vi "Set Torque Setpoint.vi"(8 "error in (no error)":errorcluster, 10 "current (A)":dbl, 11 "NI_Robotics_KUKA youBot Arm Motor_EtherCAT in":refnum<class "NI_Robotics_KUKA youBot Arm Motor_EtherCAT.lvclass">) -> (0 "error out":errorcluster, 3 "NI_Robotics_KUKA youBot Arm Motor_EtherCAT out":refnum<class "NI_Robotics_KUKA youBot Arm Motor_EtherCAT.lvclass">)   [LabVIEW 2017, in "NI_Robotics_KUKA youBot Host.lvlib" / "NI_Robotics_KUKA youBot Arm Motor_EtherCAT.lvclass"]
uses:
  <vilib>/robotics/KUKA youBot/Motor/Arm Motor EtherCAT/NI_Robotics_KUKA youBot Arm Motor_EtherCAT.lvclass
  <vilib>/robotics/KUKA youBot/Motor/Arm Motor EtherCAT/NI_Robotics_KUKA youBot Arm Motor_EtherCAT.lvclass/NI_Robotics_KUKA youBot Arm Motor_EtherCAT.ctl
  <vilib>/robotics/KUKA youBot/EtherCAT/Control Mode.ctl
  <vilib>/robotics/KUKA youBot/NI_Robotics_KUKA youBot Host.lvlib
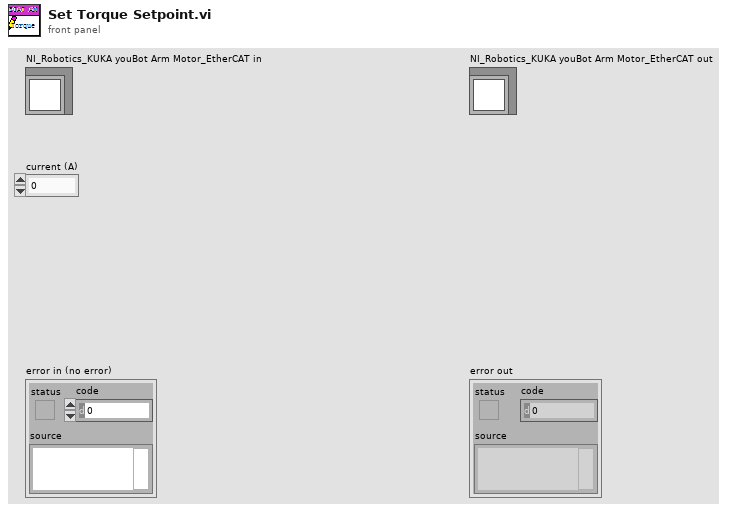
[diagram p1: front panel]
types:
  T1 = typedef "NI_Robotics_KUKA youBot Host.lvlib/Control Mode.ctl" = u8
  T2 = typedef "NI_Robotics_KUKA youBot Host.lvlib/Motor Slave Info.ctl" = cluster{"controller mode var":refnum<k21>, "reference var":refnum<k21>, "current var":refnum<k21>, "velocity var":refnum<k21>, "position var":refnum<k21>, "status var":refnum<k21>, "valid":bool, "status var type":enum16{"Int16", "Int32"}, "nodeAddr":u16, "masterHdl":T3}
  T3 = typedef "NI_Robotics_KUKA youBot Host.lvlib/Mater Handler.ctl" = i32
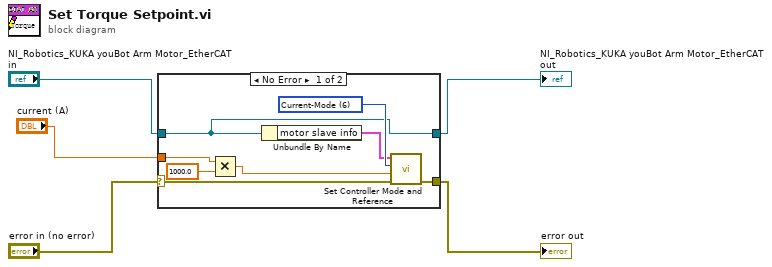
[diagram p0: block diagram]
diagram:
  n1 = case shown="No Error" "error in (no error)" {
    selector: "error in (no error)" -> [w9 w14]
    tunnel: [w11 w14] -> w2
    tunnel: [w10 w15] -> w4
    tunnel: "NI_Robotics_KUKA youBot Arm Motor_EtherCAT in" -> [w10 w15]
    tunnel: "current (A)" -> [w8 _]
    frame No Error {
      w13 = T1 6 items=["Motor Stop", "Positioning-Mode", "Velocity-Mode", "no more action", "set position to reference", "PWM-Mode", "Current-Mode", "Initialize"] ("controller mode")
      n2 = Multiply(x=w8, y=1000.0) -> (x*y=w6:dbl)
      n3 = Unbundle By Name(w10) -> ("motor slave info"=w12:T2)
      n4 = call <vilib>:"Set Controller Mode and Reference.vi"("error in (no error)"=w9, "reference"=w6, "controller mode"=w13, "motor slave info in"=w12) -> ("error out"=w11:errorcluster)  [unwired: 5 in, 2 out]
    }
    frame Error {
    }
  }
  "error out" <- w2
  "NI_Robotics_KUKA youBot Arm Motor_EtherCAT out" <- w4
